vi "_PluginLoader_LoadPlugins.vi"(8 "error in (no error)":errorcluster, 11 "_PluginLoader in":refnum<class "_PluginLoader.lvclass">) -> (0 "error out":errorcluster, 3 "_PluginLoader out":refnum<class "_PluginLoader.lvclass">)   [LabVIEW 2014, in "_PluginLoader.lvclass"]
uses:
  _PluginLoader.lvclass
  _PluginLoader.lvclass/_PluginLoader.ctl
  GCMPlugin/GCMPlugin.lvclass
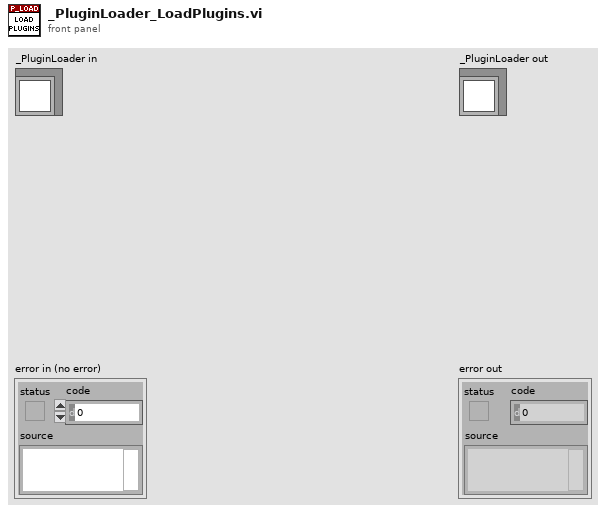
[diagram p1: front panel]
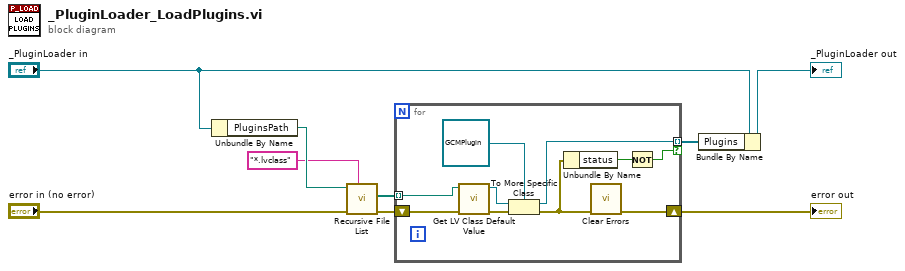
[diagram p0: block diagram]
diagram:
  n1 = Unbundle By Name("_PluginLoader in") -> ("PluginsPath"=w5:path)
  n2 = call <vilib>:"Recursive File List.vi"("pattern"="*.lvclass", "error in (no error)"="error in (no error)", "Folder Path"=w5) -> ("error out"=w2:errorcluster, "All Files in Dir"=w3:path[])  [unwired: 4 in, 3 out]
  n3 = for {
    tunnel: w3 -> [w19] mode=indexing
    tunnel: [w14] -> w1 mode=indexing if=w10
    shift-right: [w13] -> w8
    shift-left: w2 -> [w16]
    n4 = call <vilib>:"Get LV Class Default Value.vi"("error in (no error)"=w16, "class path"=w19) -> ("error out"=w17:errorcluster, "object"=w18:refnum<class>)  [unwired: 8 in]
    n5 = To More Specific Class(target class=refnum<class "GCMPlugin.lvclass"> refnum ("_LVCMPlugin.lvclass"), reference=w18, error in=w17) -> (specific class reference=w14:refnum<class "GCMPlugin.lvclass">, error out=w12:errorcluster)
    n6 = Unbundle By Name(w12) -> ("status"=w11:bool)
    n7 = call <vilib>:"Clear Errors.vi"("error in (no error)"=w12) -> ("error out"=w13:errorcluster)  [unwired: 5 in, 1 out]
    n8 = Not(x=w11) -> (.not. x?=w10:bool)
  }
  "error out" <- w8
  n9 = Bundle By Name(cluster="_PluginLoader in", "Plugins"=w1) -> (→"_PluginLoader out":refnum<class "_PluginLoader.lvclass">)
